vi "WhileLoop-Demo3.vi"() -> ()   [LabVIEW 2018]
panel:
  out "Triggered":bool
  in  "Threshold":dbl
  in  "Slide":dbl(slide) scale=0.0..10.0
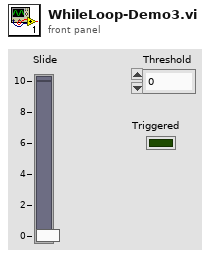
[diagram p1: front panel]
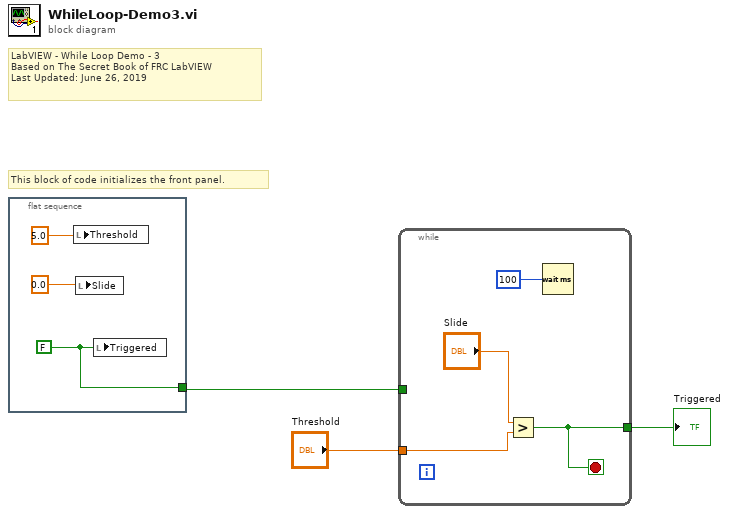
[diagram p0: block diagram]
diagram:
  # "LabVIEW - While Loop Demo - 3\nBased on The Secret Book of FRC LabVIEW\nLast Updated: June 26, 2019"
  # "This block of code initializes the front panel."
  n1 = flat-sequence {
    tunnel: [w5] -> w3
    frame #0 {
      w5 = FALSE ("Triggered")
      n2 = local write "Threshold"(5.0 ("Threshold")) -> ()
      n3 = local write "Slide"(0.0 ("Slide")) -> ()
      n4 = local write "Triggered"(w5) -> ()
    }
  }
  n5 = while {
    tunnel: w3 -> [_]
    tunnel: "Threshold" -> [w10]
    tunnel: [w8] -> w1
    stop <- w8 stop-if-true
    n6 = Greater?(x="Slide", y=w10) -> (0:w8:bool)
    n7 = Wait (ms)(milliseconds to wait=u32 100 ("millisecond timer value")) -> ()  [unwired: 1 out]
  }
  "Triggered" <- w1
